vi "Remove Device From Map.vi"(7 "Device":string, 8 "error in (no error)":errorcluster, 11 "Configuration in":refnum<class "Configuration.lvclass">) -> (0 "error out":errorcluster, 3 "Configuration out":refnum<class "Configuration.lvclass">)   [LabVIEW 2023, in "Configuration.lvlib" / "Configuration.lvclass"]
uses:
  Library/Configuration.lvclass
  Library/Configuration.lvclass/Configuration.ctl
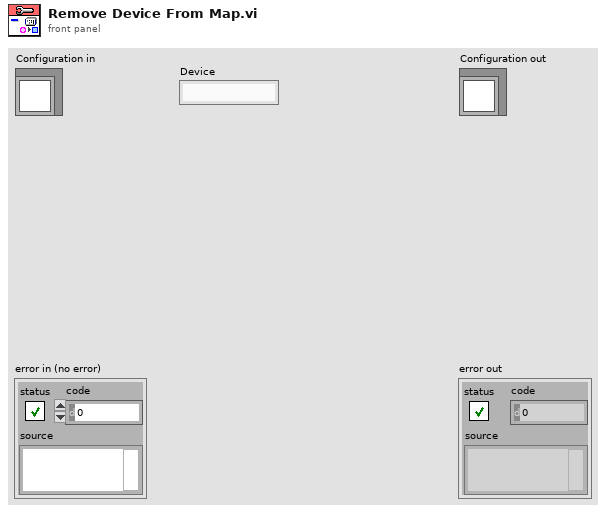
[diagram p1: front panel]
types:
  T1 = typedef "Configuration.lvlib/Configuration.lvclass/Definitions.ctl" = map{string, T2}
  T2 = typedef "Configuration.lvlib/Configuration.lvclass/Config.ctl" = map{string, string}
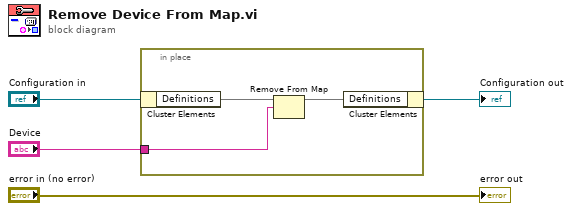
[diagram p0: block diagram]
diagram:
  n1 = in-place {
    in-place-border: "Device" -> [w5]
    n2 = in-place-cluster #1("Configuration in") -> ("Definitions"=w7:T1)
    n3 = Remove From Map(10:w5, 11:w7) -> (3:w6:T1)  [unwired: 2 out]
    n4 = in-place-cluster #1("Definitions"=w6) -> (→"Configuration out":refnum<class "Configuration.lvclass">)
  }
  "error out" <- "error in (no error)"
